vi "solar_msg Q Release.vi"(8 "error in (no error)":errorcluster, 9 "Force Destroy? (F)":bool, 11 "Queue":refnum<queue>) -> (0 "error out":errorcluster, 2 "MSGs":cluster{"MSG":string, "DATA":variant}[](array[cluster]), 3 "Queue Name":string)   [LabVIEW 2018]
doc: "This releases a queue reference. <b>Force Destroy?</b> destroys all instances of the queue."
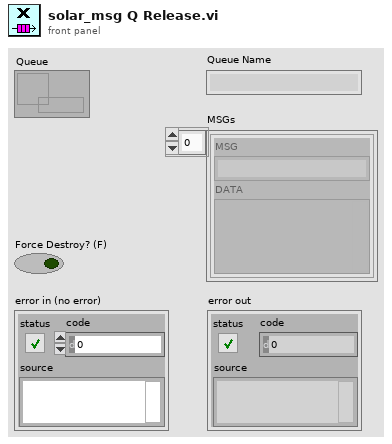
[diagram p1: front panel]
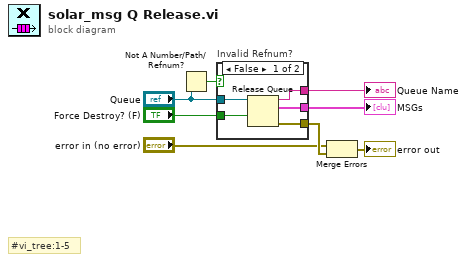
[diagram p0: block diagram]
diagram:
  # "#vi_tree:1-5"
  n1 = Not A Number/Path/Refnum?(number/path/refnum="Queue") -> (NaN/Path/Refnum?=w6:bool)
  n2 = case "Invalid Refnum?" shown="False" w6 {
    tunnel: [w13 _] -> w8
    tunnel: "Force Destroy? (F)" -> [w12 _]
    tunnel: [w11 _] -> w1
    tunnel: [w10 _] -> w2
    tunnel: "Queue" -> [w9 _]
    frame False {
      n3 = Release Queue(queue=w9, force destroy? (F)=w12) -> (queue name=w11:string, remaining elements=w10:cluster{"MSG":string, "DATA":variant}[], error out=w13:errorcluster)  [unwired: 1 in]
    }
    frame True {
    }
  }
  "Queue Name" <- w1
  "MSGs" <- w2
  n4 = Merge Errors("error in (no error)", w8) -> (→"error out":errorcluster)
